vi "ChangeInheritance_DEPRECATED.vi"(0 "LibWriter":refnum<class "LibWriter.lvclass">, 1 "LvClass":refnum<vi>, 2 "NewBaseClass(Empty=ConvertClassToBaseClass)":path=path "C:/Documents and Settings/Micke/Skrivbord/My Computer/B_class/B.lvclass", 5 "error in (no error)":errorcluster) -> (14 "LibWriter":refnum<class "LibWriter.lvclass">, 19 "error out":errorcluster)   [LabVIEW 2014]
uses:
  <resource>/Framework/Providers/Open_GDS/ClassProviders/LibProvider_BaseClassInterface/LibWriter_class/ClassWriter_class/LibWriter.lvclass
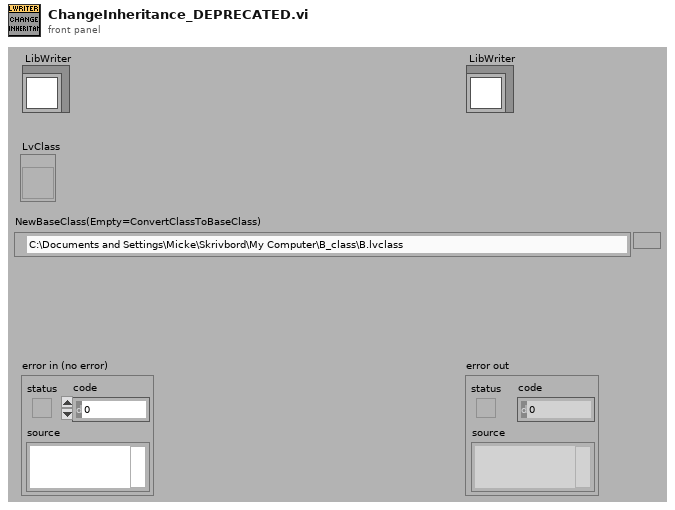
[diagram p1: front panel]
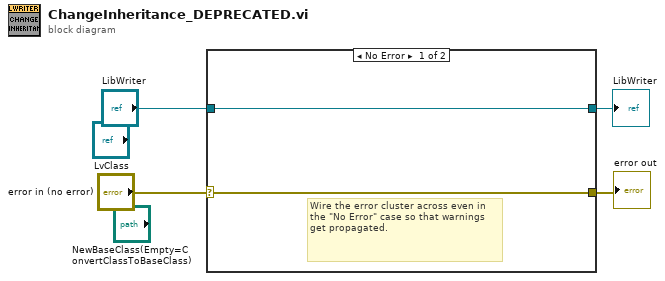
[diagram p0: block diagram]
diagram:
  n1 = case shown="No Error" "error in (no error)" {
    selector: "error in (no error)" -> [w5 w8]
    tunnel: [w5 w8] -> w3
    tunnel: [w6 w7] -> w1
    tunnel: "LibWriter" -> [w6 w7]
    frame No Error {
      # "Wire the error cluster across even in the \"No Error\" case so that warnings get propagated."
    }
    frame Error {
    }
  }
  "error out" <- w3
  "LibWriter" <- w1
